vi "UI - By List.vi"(5 "Term (Methods)":string="Methods", 7 "Msg Chain":string, 8 "error in (no error)":errorcluster {"code" format="Error %.0f"}, 10 "UI Docs":refnum<class "GUI Documentation.lvclass">[](array[class]), 11 "VIDoc Printer - Confluence In":refnum<class "VIDoc Printer - Confluence.lvclass">) -> (0 "error out":errorcluster {"code" format="Error %.0f"}, 3 "VIDoc Printer - Confluence Out":refnum<class "VIDoc Printer - Confluence.lvclass">)   [LabVIEW 2023, in "VIDoc Printer - Confluence.lvlib" / "VIDoc Printer - Confluence.lvclass"]
uses:
  VIDoc Printer - Confluence.lvclass
  VIDoc Printer - Confluence.lvclass/VIDoc Printer - Confluence.ctl
  Confluence Formatting/Confluence Formatting.lvlib
  Confluence Formatting/Types/Format Combo Box.ctl
  Printer/VIDoc Printer.lvclass
  Parsing/GUI Documentation/GUI Documentation.lvclass
  UI Interaction/UI Interaction.lvclass
  Types/VI Method Types.ctl
  C:/projects/DMC/Tooling/Git-Action-Service/Source/Documentation Generation/Printers/Printer/VIDoc Printer.lvclass
  C:/projects/DMC/Tooling/Git-Action-Service/Source/Documentation Generation/Printers/Confluence Printer/VIDoc Printer - Confluence.lvclass
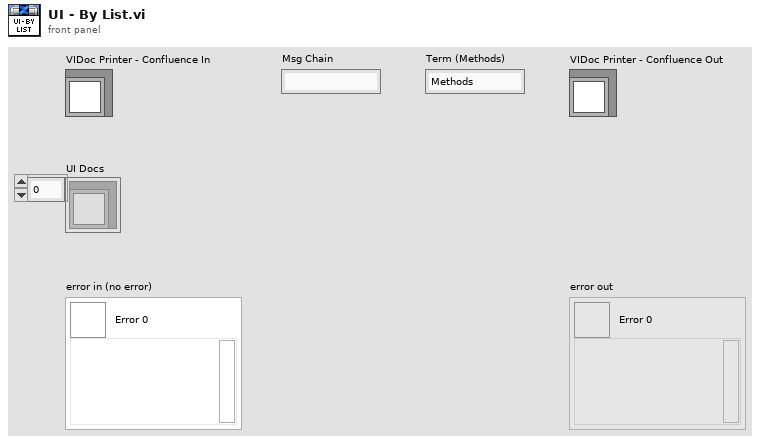
[diagram p1: front panel]
types:
  T1 = typedef "Confluence Formatting.lvlib/Format Combo Box.ctl" = string
  T2 = typedef "VIDoc Printer.lvlib/Printer Settings.lvclass/VI Settings.ctl" = cluster{"Memory":bool, "By Folder":bool, "By Tree":bool, "By List":bool, "Methods":bool, "Method Options":cluster{"Front Panels":bool, "Options":bool, "Controls":bool}, "List Detail Level":T3, "Methods Detail Level":T3, "Controls Detail Level":T3}
  T3 = typedef "VIDoc Printer.lvlib/Printer Settings.lvclass/Detail Level Enum.ctl" = enum16{"None", "Minimal", "Standard", "Full"}
  T4 = typedef "VIDoc Printer.lvlib/Printer Settings.lvclass/Bookmark Options.ctl" = cluster{"Bookmarks as New Line in VI Descriptions":bool, "Unique Bookmark Tags Only":bool, "Include Tag and Text":bool}
  T5 = typedef "VIDoc Printer - Confluence.lvlib/VIDoc Printer - Confluence.lvclass/VI Method Types.ctl" = enum16{"Library", "Class", "Interface", "LLB", "UI", "List"}
  T6 = typedef "VIDoc Parsing.lvlib/Method Spec Cluster.ctl" = cluster{"VI Type Ext":T7, "Name":string, "Path":path, "Get Conpane Image":T8, "Description":string, "Get Library Access Scope":enum32{"invalid scope", "public", "private", "protected", "community"}, "Dispatch":T9, "ContainsCompiledCode":bool, "Exec.IsReentrant":bool, "Exec.ReentrancyType":enum16{"Share clones between instances", "Preallocate clone for each instance"}, "ExecInlining":bool, "ExecInlineIfPossible":bool, "Auto Err Handling":bool, "CodeComplexity":sgl, "Bookmark Tags":string[], "Control VI Type":enum32{"not a control VI", "control", "typedef", "strict typedef"}, "Controls":T10[], "VI Type":enum32{"invalid VI type", "Standard VI", "Control VI", "Global VI", "Polymorphic VI", "Configuration VI", "SubSystem", "Facade VI", "Method VI", "Statechart Diagram VI"}, "Minimum Size":T12, "Front Panel Window:Title":string, "Front Panel Window:Behavior":enum32{"Invalid", "Default", "Floating", "Floating/Auto-Hide", "Modal"}, "Front Panel Window:Closeable":bool, "Must Override":bool, "Must Use Parent Implementation":bool, "VI Icon":T8, "Front Panel":T8, "History:Revision Number":u32, "Metrics:Total Data Size":u32, "Execution:Allow Debugging":bool, "Execution:Preferred Exec System":enum32{"invalid execution system", "user interface", "standard", "instrument i/o", "data acquisition", "other 1", "other 2", "same as caller"}, "Execution:Priority":enum32{"invalid priority", "background priority", "normal priority", "above normal priority", "high priority", "time critical priority", "subroutine"}, "BM Tag Text":string[], "Block Diagram":T8, "Structure Tree":T13[]}
  T7 = typedef "VIDoc Parsing.lvlib/VI Type Extended Enum.ctl" = enum16{"Unknown", "Class Method", "Class Accessor Get", "Class Accessor Set", "Class Control", "Library Method", "Library Control", "VI", "Control"}
  T8 = typedef "imagedata.ctl" = cluster{"image type":i32, "image depth":i32, "image":u8[], "mask":u8[], "colors":u32[], "Rectangle":cluster{"left":i16, "top":i16, "right":i16, "bottom":i16}}
  T9 = typedef "VIDoc Parsing.lvlib/Class Dispatch Type Enum.ctl" = enum16{"None", "Static", "Dynamic"}
  T10 = typedef "VIDoc Parsing.lvlib/Controls Info Cluster.ctl" = cluster{"Name":string, "Description":string, "Data Type":string, "Tip Strip":string, "UID":i32, "Image Data":T8, "ToggleKeyBind":T11, "Raw Label":string, "Raw Caption":string}
  T11 = typedef "LVKeyTypeDef.ctl" = cluster{"Focus":bool, "Control":bool, "Shift":bool, "Key":string}
  T12 = typedef "LVPointTypeDef.ctl" = cluster{"Horizontal":i16, "Vertical":i16}
  T13 = typedef "VIDoc Parsing.lvlib/Structure Reporter.lvlib/Tree Cluster.ctl" = cluster{"Object Class Name":string, "Labels":string[], "Child Tag":string, "Item Indent":i32, "Child Only?":bool, "Glyph Index":i32}
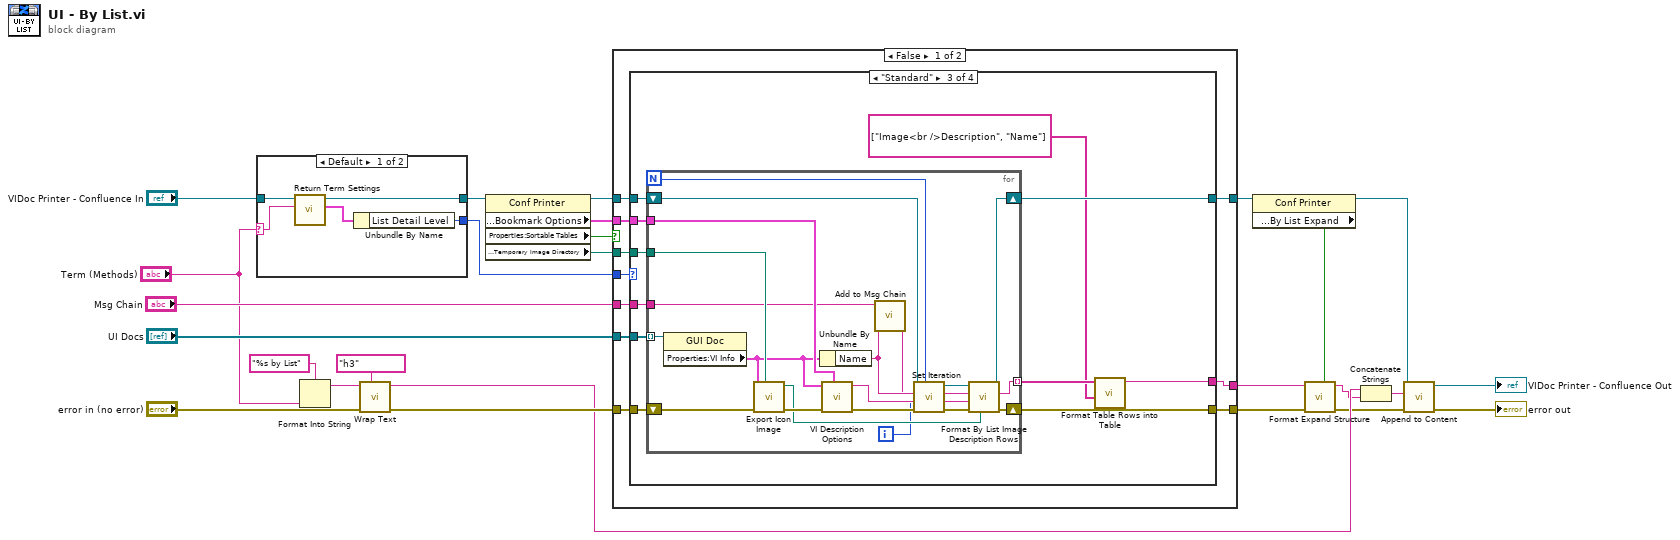
[diagram p0: block diagram]
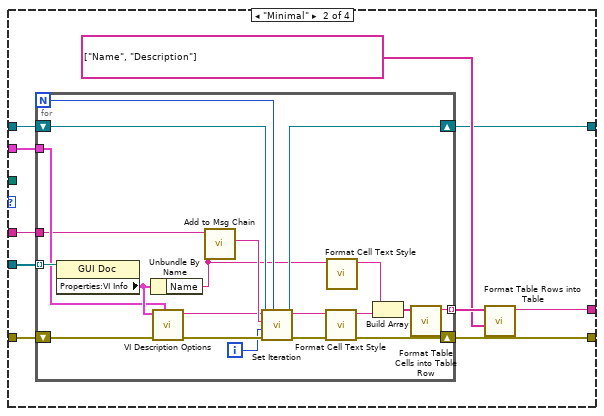
[diagram p3: hidden frame]
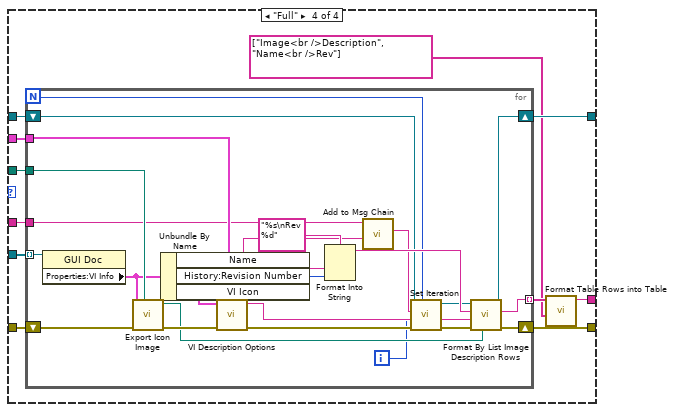
[diagram p4: hidden frame]
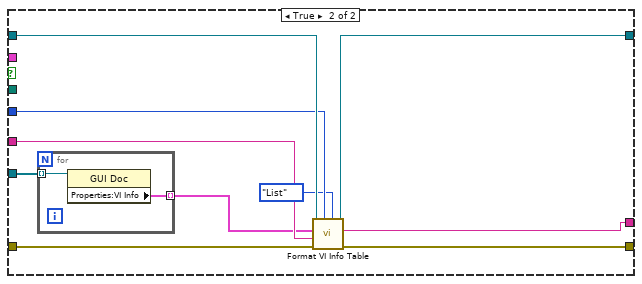
[diagram p5: hidden frame]
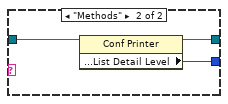
[diagram p6: hidden frame]
diagram:
  n1 = case shown="Default" "Term (Methods)" {
    selector: "Term (Methods)" -> [w29 _]
    tunnel: "VIDoc Printer - Confluence In" -> [w31 w34]
    tunnel: [w30 w33] -> w10
    tunnel: [w27 w32] -> w9
    frame Default {
      n2 = call "Return Term Settings.vi"("Term"=w29, "Printer in"=w31) -> ("Term Settings"=w28:T2, "Printer out"=w30:refnum<class "VIDoc Printer - Confluence.lvclass">)  [unwired: 6 in, 2 out]
      n3 = Unbundle By Name(w28) -> ("List Detail Level"=w27:T3)
    }
    frame "Methods" {
      n4 = property class="Conf Printer"(reference=w34) -> (reference out=w33:refnum<class "VIDoc Printer - Confluence.lvclass">, "Properties:Settings:VI Members:List Detail Level"=w32:T3)  [unwired: 1 in, 1 out]
    }
  }
  n5 = Format Into String(format string="%s by List", "Term (Methods)") -> (resulting string=w20:string)  [unwired: 2 in, 1 out]
  n6 = call "Wrap Text.vi"("Formatting"=T1 "h3", "Error in"="error in (no error)", "String"=w20) -> ("Error out"=w19:errorcluster, "Wrapped String"=w13:string)  [unwired: 7 in]
  n7 = property class="Conf Printer"(reference=w10) -> (reference out=w16:refnum<class "VIDoc Printer - Confluence.lvclass">, "Properties:Settings:Formatting Options:Bookmark Options"=w11:T4, "Properties:Sortable Tables"=w3:bool, "Properties:Temporary Image Directory"=w2:path)  [unwired: 1 in, 1 out]
  n8 = case shown="False" w3 {
    tunnel: w19 -> [w44 w149]
    tunnel: [w43 w148] -> w18
    tunnel: "UI Docs" -> [w42 w141]
    tunnel: w16 -> [w41 w146]
    tunnel: [w40 w145] -> w15
    tunnel: w2 -> [w39 _]
    tunnel: "Msg Chain" -> [w38 w142]
    tunnel: w11 -> [w37 _]
    tunnel: w9 -> [w36 w144]
    tunnel: [w35 w147] -> w7
    frame False {
      n9 = case shown="\"Standard\"" w36 {
        tunnel: w44 -> [w46 w54 w83 w114]
        tunnel: [w46 w51 w77 w108] -> w43
        tunnel: w42 -> [_ w56 w85 w116]
        tunnel: w37 -> [_ w55 w84 w115]
        tunnel: [_ w52 w79 w110] -> w35
        tunnel: w41 -> [w45 w49 w81 w112]
        tunnel: [w45 w48 w80 w111] -> w40
        tunnel: w39 -> [_ _ w82 w113]
        tunnel: w38 -> [_ w47 w75 w106]
        frame "None", Default {
        }
        frame "Minimal" {
          n10 = for {
            N -> [w64]
            tunnel: w56 -> [w74] mode=indexing
            tunnel: w55 -> [w72]
            shift-right: [w67] -> w51
            shift-left: w54 -> [w71]
            tunnel: [w69] -> w53 mode=indexing
            shift-right: [w65] -> w48
            shift-left: w49 -> [w66]
            tunnel: w47 -> [w62]
            i -> [w63]
            n11 = property class="GUI Doc"(reference=w74) -> ("Properties:VI Info"=w73:T6)  [unwired: 1 in, 2 out]
            n12 = Unbundle By Name(w73) -> ("Name"=w59:string)
            n13 = call "VI Description Options.vi"("Bookmark Options"=w72, "Error in"=w71, "VI Info"=w73) -> ("Error out"=w68:errorcluster, "Description"=w58:string)  [unwired: 7 in]
            n14 = call "Add to Msg Chain.vi"("New"=w59, "Msg Chain in"=w62) -> ("Msg Chain out"=w61:string)  [unwired: 9 in]
            n15 = call "Set Iteration.vi"("Progress Max"=w64, "error in (no error)"=w68, "Progress Value"=w63, "Message (No Message Update)"=w61, "VIDoc Printer In"=w66) -> ("error out"=w67:errorcluster, "VIDoc Printer Out"=w65:refnum<class "VIDoc Printer - Confluence.lvclass">)  [unwired: 4 in, 1 out]
            n16 = call "Format Cell Text Style.vi"("String"=w58) -> ("Formatted Text"=w57:string)  [unwired: 9 in, 1 out]
            n17 = call "Format Cell Text Style.vi"("String"=w59) -> ("Formatted Text"=w60:string)  [unwired: 9 in, 1 out]
            n18 = Build Array(w60, w57) -> (w70:string[])
            n19 = call "Format Table Cells into Table Row.vi"("Table Cells"=w70) -> ("Table Row Text"=w69:string)  [unwired: 10 in]
          }
          n20 = call "Format Table Rows into Table.vi"("Table Headers"=string[] ["Name", "Description"], "Table Rows"=w53) -> ("Table Text"=w52:string)  [unwired: 9 in]
        }
        frame "Standard" {
          n21 = for {
            N -> [w90]
            tunnel: w85 -> [w105] mode=indexing
            tunnel: w84 -> [w104]
            shift-right: [w99] -> w77
            shift-left: w83 -> [w102]
            tunnel: w82 -> [w103]
            shift-right: [w98] -> w80
            shift-left: w81 -> [w92]
            tunnel: [w95] -> w78 mode=indexing
            tunnel: w75 -> [w88]
            i -> [w89]
            n22 = property class="GUI Doc"(reference=w105) -> ("Properties:VI Info"=w100:T6)  [unwired: 1 in, 2 out]
            n23 = call "Export Icon Image.vi"("Temporary Image Directory"=w103, "Error in"=w102, "VI Info"=w100) -> ("Error out"=w101:errorcluster, "Image Path"=w96:path)  [unwired: 7 in]
            n24 = Unbundle By Name(w100) -> ("Name"=w87:string)
            n25 = call "VI Description Options.vi"("Bookmark Options"=w104, "Error in"=w101, "VI Info"=w100) -> ("Error out"=w94:errorcluster, "Description"=w97:string)  [unwired: 7 in]
            n26 = call "Add to Msg Chain.vi"("New"=w87, "Msg Chain in"=w88) -> ("Msg Chain out"=w86:string)  [unwired: 9 in]
            n27 = call "Set Iteration.vi"("Progress Max"=w90, "error in (no error)"=w94, "Progress Value"=w89, "Message (No Message Update)"=w86, "VIDoc Printer In"=w92) -> ("error out"=w93:errorcluster, "VIDoc Printer Out"=w91:refnum<class "VIDoc Printer - Confluence.lvclass">)  [unwired: 4 in, 1 out]
            n28 = call "Format By List Image Description Rows.vi"("Image"=w96, "error in (no error)"=w93, "Description"=w97, "Name"=w87, "VIDoc Printer - Confluence In"=w91) -> ("error out"=w99:errorcluster, "Table Rows Text"=w95:string, "VIDoc Printer - Confluence Out"=w98:refnum<class "VIDoc Printer - Confluence.lvclass">)  [unwired: 3 in, 1 out]
          }
          n29 = call "Format Table Rows into Table.vi"("Table Headers"=string[] ["Image<br />Description", "Name"], "Table Rows"=w78) -> ("Table Text"=w79:string)  [unwired: 9 in]
        }
        frame "Full" {
          n30 = for {
            N -> [w121]
            tunnel: w116 -> [w139] mode=indexing
            tunnel: w115 -> [w138]
            shift-right: [w133] -> w108
            shift-left: w114 -> [w136]
            tunnel: w113 -> [w137]
            shift-right: [w132] -> w111
            shift-left: w112 -> [w123]
            tunnel: [w129] -> w109 mode=indexing
            tunnel: w106 -> [w119]
            i -> [w120]
            n31 = property class="GUI Doc"(reference=w139) -> ("Properties:VI Info"=w134:T6)  [unwired: 1 in, 2 out]
            n32 = call "Export Icon Image.vi"("Temporary Image Directory"=w137, "Error in"=w136, "VI Info"=w134) -> ("Error out"=w135:errorcluster, "Image Path"=w130:path)  [unwired: 7 in]
            n33 = Unbundle By Name(w134) -> ("Name"=w118:string, "History:Revision Number"=w127:u32)  [unwired: 1 out]
            n34 = call "VI Description Options.vi"("Bookmark Options"=w138, "Error in"=w135, "VI Info"=w134) -> ("Error out"=w125:errorcluster, "Description"=w131:string)  [unwired: 7 in]
            n35 = Format Into String(format string="%s\nRev %d", w118, w127) -> (resulting string=w126:string)  [unwired: 2 in, 1 out]
            n36 = call "Add to Msg Chain.vi"("New"=w118, "Msg Chain in"=w119) -> ("Msg Chain out"=w117:string)  [unwired: 9 in]
            n37 = call "Set Iteration.vi"("Progress Max"=w121, "error in (no error)"=w125, "Progress Value"=w120, "Message (No Message Update)"=w117, "VIDoc Printer In"=w123) -> ("error out"=w124:errorcluster, "VIDoc Printer Out"=w122:refnum<class "VIDoc Printer - Confluence.lvclass">)  [unwired: 4 in, 1 out]
            n38 = call "Format By List Image Description Rows.vi"("Image"=w130, "error in (no error)"=w124, "Description"=w131, "Name"=w126, "VIDoc Printer - Confluence In"=w122) -> ("error out"=w133:errorcluster, "Table Rows Text"=w129:string, "VIDoc Printer - Confluence Out"=w132:refnum<class "VIDoc Printer - Confluence.lvclass">)  [unwired: 3 in, 1 out]
          }
          n39 = call "Format Table Rows into Table.vi"("Table Headers"=string[] ["Image<br />Description", "Name<br />Rev"], "Table Rows"=w109) -> ("Table Text"=w110:string)  [unwired: 9 in]
        }
      }
    }
    frame True {
      n40 = for {
        tunnel: w141 -> [w151] mode=indexing
        tunnel: [w150] -> w140 mode=indexing
        n41 = property class="GUI Doc"(reference=w151) -> ("Properties:VI Info"=w150:T6)  [unwired: 1 in, 2 out]
      }
      n42 = call "Format VI Info Table.vi"("Type"=VI_Method_Types."List", "Methods"=w144, "Error in"=w149, "Msg Chain"=w142, "VI Info Array"=w140, "VIDoc Printer - Confluence In"=w146) -> ("Error out"=w148:errorcluster, "Table String"=w147:string, "VIDoc Printer - Confluence Out"=w145:refnum<class "VIDoc Printer - Confluence.lvclass">)  [unwired: 3 in]
    }
  }
  n43 = property class="Conf Printer"(reference=w15) -> (reference out=w5:refnum<class "VIDoc Printer - Confluence.lvclass">, "Properties:Expand?:VI:By List Expand"=w4:bool)  [unwired: 1 in, 1 out]
  n44 = call "Format Expand Structure.vi"("Enable? (T)"=w4, "Error in"=w18, "Content"=w7) -> ("Error out"=w8:errorcluster, "Expand String"=w6:string)  [unwired: 7 in]
  n45 = Concatenate Strings(w13, w6) -> (w14:string)
  n46 = call "Append to Content.vi"("error in (no error)"=w8, "Content"=w14, "VIDoc Printer - Confluence In"=w5) -> ("error out"=→"error out":errorcluster, "VIDoc Printer - Confluence Out"=→"VIDoc Printer - Confluence Out":refnum<class "VIDoc Printer - Confluence.lvclass">)  [unwired: 7 in]
